vi "Read Actor Index.vi"(11 "Actor in":refnum<class "Actor.lvclass">) -> (2 "Actor Index":i32)   [LabVIEW 2025, in "jettl.lvlib" / "Actor.lvclass"]
uses:
  Actor.lvclass
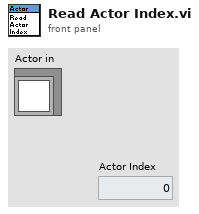
[diagram p1: front panel]
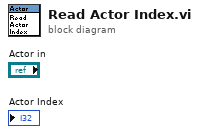
[diagram p0: block diagram]
diagram:
